vi "Hex to Dec.vi"(0 "Bz":string) -> (18 "decimal":u8, 20 "Checkbox":bool, 21 "Checkbox 2":bool, 22 "Checkbox 3":bool, 23 "Checkbox 4":bool, 24 "Checkbox 5":bool, 25 "Checkbox 6":bool, 26 "Checkbox 7":bool, 27 "Checkbox 8":bool)   [LabVIEW 2020]
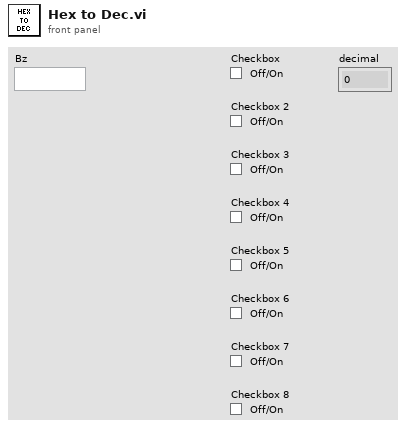
[diagram p1: front panel]
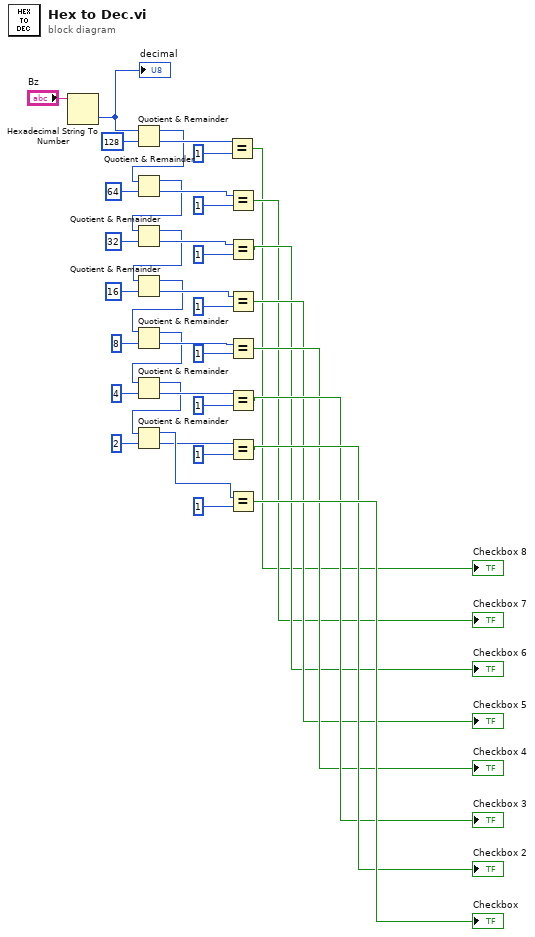
[diagram p0: block diagram]
diagram:
  n1 = Hexadecimal String To Number(string="Bz") -> (number=w30:u32)  [unwired: 2 in, 1 out]
  "decimal" <- w30
  n2 = Quotient & Remainder(x=w30, y=u8 128) -> (x-y*floor(x/y)=w10:u32, floor(x/y)=w22:u32)
  n3 = Quotient & Remainder(x=w10, y=u8 64) -> (x-y*floor(x/y)=w11:u32, floor(x/y)=w28:u32)
  n4 = Quotient & Remainder(x=w11, y=u8 32) -> (x-y*floor(x/y)=w12:u32, floor(x/y)=w23:u32)
  n5 = Quotient & Remainder(x=w12, y=u8 16) -> (x-y*floor(x/y)=w13:u32, floor(x/y)=w24:u32)
  n6 = Quotient & Remainder(x=w13, y=u8 8) -> (x-y*floor(x/y)=w14:u32, floor(x/y)=w25:u32)
  n7 = Quotient & Remainder(x=w14, y=u8 4) -> (x-y*floor(x/y)=w15:u32, floor(x/y)=w26:u32)
  n8 = Quotient & Remainder(x=w15, y=u8 2) -> (x-y*floor(x/y)=w29:u32, floor(x/y)=w27:u32)
  n9 = Equal?(x=w22, y=u8 1) -> (x = y?=→"Checkbox 8":bool)
  n10 = Equal?(x=w28, y=u8 1) -> (x = y?=→"Checkbox 7":bool)
  n11 = Equal?(x=w23, y=u8 1) -> (x = y?=→"Checkbox 6":bool)
  n12 = Equal?(x=w24, y=u8 1) -> (x = y?=→"Checkbox 5":bool)
  n13 = Equal?(x=w25, y=u8 1) -> (x = y?=→"Checkbox 4":bool)
  n14 = Equal?(x=w26, y=u8 1) -> (x = y?=→"Checkbox 3":bool)
  n15 = Equal?(x=w27, y=u8 1) -> (x = y?=→"Checkbox 2":bool)
  n16 = Equal?(x=w29, y=u8 1) -> (x = y?=→"Checkbox":bool)
